vi "Emergency Stop.vi"(8 "error in (no error)":errorcluster, 10 "Wheel (-1: all)":i32, 11 "FW Arduino Control in":refnum<class "FW Arduino Control.lvclass">) -> (0 "error out":errorcluster, 3 "FW Arduino Control out":refnum<class "FW Arduino Control.lvclass">)   [LabVIEW 2021, in "FW Arduino Control.lvclass"]
uses:
  FW Arduino Control.lvclass
  C:/Development/prime/Prime-RIMAS/Filter Wheel/Filter Wheel Object/Filter Wheel.lvclass
  Filter Wheel Object/Filter Wheel.lvclass
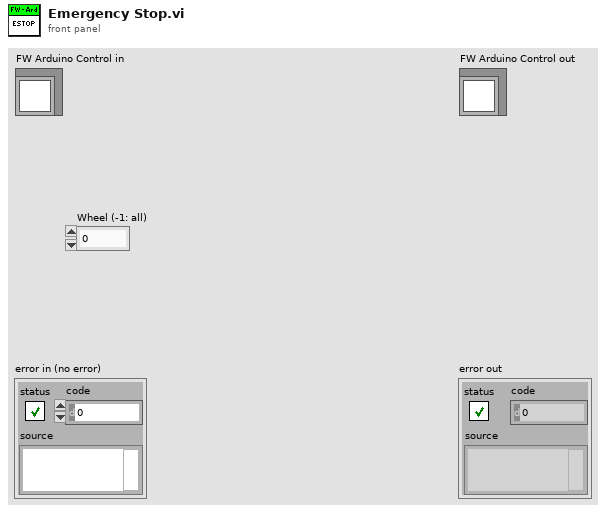
[diagram p1: front panel]
types:
  T1 = typedef "Filter Wheel.lvclass/Filter Wheel configuration.ctl" = cluster{"Num Wheels":i32, "Filters":T2[], "Invalid Combinations":i32[][], "Addr":refnum<visa-resource-name>, "Name":string, "Simulate":bool, "Homing Parameters":T3, "Default Speed":u16}
  T2 = typedef "Filter Wheel.lvclass/Filter Wheel Details.ctl" = cluster{"Names":string[], "Relative Position":i32[], "Wheel Name":string}
  T3 = typedef "Filter Wheel Arduino Homing cluster.ctl" = cluster{"Direction (F: CW)":bool, "Speed":i32, "Accel":i32, "Min Distance":i32, "Short Leg":i32, "Error Cnts":i32}
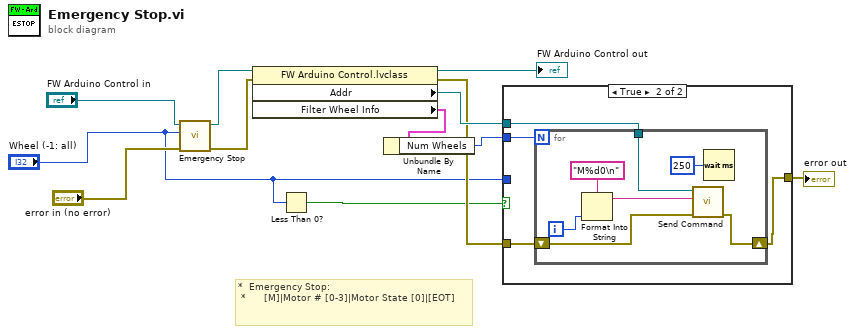
[diagram p0: block diagram]
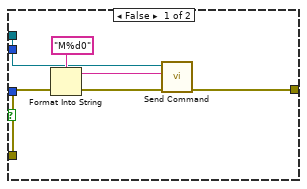
[diagram p2: hidden frame]
diagram:
  # "*  Emergency Stop:\n *      [M]|Motor # [0-3]|Motor State [0]|[EOT]"
  n1 = call-parent "Emergency Stop.vi"("error in (no error)"="error in (no error)", "Wheel (-1: all)"="Wheel (-1: all)", "Filter Wheel in"="FW Arduino Control in") -> ("error out"=w3:errorcluster, "Filter Wheel out"=w9:refnum<class "FW Arduino Control.lvclass">)  [unwired: 7 in]
  n2 = property class="FW Arduino Control.lvclass"(reference=w9, error in=w3) -> (reference out=→"FW Arduino Control out":refnum<class "FW Arduino Control.lvclass">, error out=w8:errorcluster, "Addr"=w10:refnum<visa-resource-name>, "Filter Wheel Info"=w2:T1)
  n3 = Less Than 0?(x="Wheel (-1: all)") -> (x < 0?=w4:bool)
  n4 = Unbundle By Name(w2) -> ("Num Wheels"=w1:i32)
  n5 = case shown="True" w4 {
    tunnel: w10 -> [w16 w22]
    tunnel: w8 -> [w15 w21]
    tunnel: [w14 w20] -> w7
    tunnel: "Wheel (-1: all)" -> [w13 _]
    tunnel: w1 -> [_ w19]
    frame False {
      n6 = Format Into String(format string="M%d0", w13) -> (resulting string=w17:string)  [unwired: 2 in, 1 out]
      n7 = call "Send Command.vi"("error in (no error)"=w15, "Command"=w17, "addr"=w16) -> ("error out"=w14:errorcluster)  [unwired: 7 in, 1 out]
    }
    frame True {
      n8 = for {
        N: w19 -> [_]
        tunnel: w22 -> [w26]
        shift-right: [w24] -> w20
        shift-left: w21 -> [w25]
        i -> [w27]
        n9 = Format Into String(format string="M%d0\n", w27) -> (resulting string=w28:string)  [unwired: 2 in, 1 out]
        n10 = call "Send Command.vi"("error in (no error)"=w25, "Command"=w28, "addr"=w26) -> ("error out"=w24:errorcluster)  [unwired: 7 in, 1 out]
        n11 = Wait (ms)(milliseconds to wait=u32 250) -> ()  [unwired: 1 out]
      }
    }
  }
  "error out" <- w7
